vi "ReadBinayFile.vi"() -> ()   [LabVIEW 2020]
panel:
  out "data":cluster{"samples":i32, "amplitude":dbl}[](array[cluster])
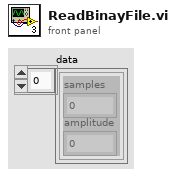
[diagram p1: front panel]
types:
  T1 = enum16{"open", "replace", "create", "open or create", "replace or create", "replace or create with confirmation"}
  T2 = enum16{"deny read/write", "deny write-only", "deny none"}
  T3 = enum16{"big-endian, network order", "native, host order", "little-endian"}
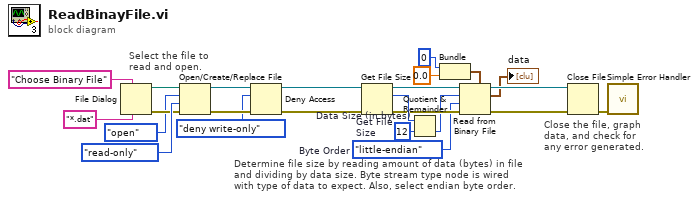
[diagram p0: block diagram]
diagram:
  w11 = T3."little-endian"  # Byte Order
  w13 = i64 12  # Data Size (in bytes)
  # "Close the file, graph data, and check for any error generated."
  # "Determine file size by reading amount of data (bytes) in file and dividing by data size. Byte stream type node is wired with type of data to expect. Also, select endian byte order."
  # "Select the file to read and open."
  n1 = File Dialog(6:"*.dat" ("pattern (all files)"), 7:"Choose Binary File" ("Prompt")) -> (0:w15:errorcluster, 3:w22:path)  [unwired: 5 in, 2 out]
  n2 = Open/Create/Replace File(file path (use dialog)=w22, error in=w15, operation (0:open)=T1."open", access (0:read/write)=enum16{"read/write", "read-only", "write-only"}."read-only") -> (refnum out=w9:refnum<file>, error out=w10:errorcluster)  [unwired: 2 in, 1 out]
  n3 = Deny Access(4:w10, 6:T2."deny write-only" ("deny mode (0:deny read/write)"), 7:w9) -> (0:w8:errorcluster, 3:w7:refnum<file>)
  n4 = Get File Size "Get File\nSize"(file=w7, error in=w8) -> (refnum out=w24:refnum<file>, size (in bytes)=w18:i64, 0:w17:errorcluster)
  n5 = Quotient & Remainder(x=w18, y=w13) -> (floor(x/y)=w12:i64)  [unwired: 1 out]
  n6 = Bundle("samples"=0, "amplitude"=0.0) -> (w2:cluster{"samples":i32, "amplitude":dbl})  [unwired: 1 in]
  n7 = Read from Binary File(5:w2, 8:w17, 9:w11, 10:w12, 11:w24) -> (0:w20:errorcluster, 2:→"data":cluster{"samples":i32, "amplitude":dbl}[], 3:w23:refnum<file>)  [unwired: 1 in, 1 out]
  n8 = Close File(refnum=w23, error in=w20) -> (error out=w19:errorcluster)  [unwired: 1 out]
  n9 = call <vilib>:"Simple Error Handler.vi"("error in (no error)"=w19) -> ()  [unwired: 4 in, 5 out]
